vi "DFD Raised Cosine Design.vi"(4 "filtering mode":T1=2 items=["No Rate Change", "Interpolation", "Decimation"], 5 "window":u16(ring) items=["None"=0, "Hanning"=1, "Hamming"=2, "Blackman-Harris"=3, "Exact Blackman"=4, "Blackman"=5, "Flat Top"=6, "4 Term B-Harris"=7, "7 Term B-Harris"=8, "Low Sidelobe"=9, "Triangular"=30], 6 "fs in [Hz]":dbl=1.0 format="%.2f", 7 "factor":i32=2, 8 "error in (no error)":errorcluster, 9 "type":enum16{"Raised Cosine", "Root Raised Cosine"}(ring), 10 "roll off":dbl=0.2, 11 "order":i32=10) -> (0 "error out":errorcluster, 2 "order out":i32, 3 "multirate filter out":T2={"mMRate_Structure"=enum."IIR", "mMRate_Mode"=0, "mMRate_Factor"=-1, "mMRate_FIRParams"={"mMRate_FIR_H"=[], "mMRate_FIR_IsNyquist?"=FALSE, "mMRate_FIR_IsSymmetric?"=FALSE}, "mMRate_CICParams"={"mMRate_CIC_#Stage"=0, "mMRate_CIC_Lag"=0, "mMRate_CIC_Type"=enum."Lowpass"}, "mMRate_Order"=0, "mMRate_Version"="2.0", "mMRate_Comments"="", "mMRate_RationalFactor"={"mMRate_L"=-1, "mMRate_M"=-1}, "mMRate_Fs"=1.0, "mMRate_Quantized?"=FALSE, "mMRate_QFilterGain"=1.0, "mMRate_CoefWl"=16, "mMRate_Scaling"={"mMRate_ScaleByPowerOf2?"=FALSE, "mMRate_ScaleType"=enum."No Norm"}, "mMRate_InputWl"=16, "mMRate_OutputWl"=16, "mMRate_OutputMode"=enum."Truncation", "mMRate_MultMode"=enum."Truncated", "mMRate_BitPruning"=FALSE, "mMRate_GainWl"=16, "mMRate_OutputFwl"=0, "mMRate_SumIwl"=0, "mMRate_InputIwl "=16, "mMRate_SumWl"=32, "mMRate_CoefIwl"=0} {"mMRate_SumWl" min=1 max=32 step=1; "mMRate_InputIwl" min=1 max=32 step=1; "mMRate_GainWl" min=1 max=32 step=1; "mMRate_OutputWl" min=1 max=32 step=1; "mMRate_InputWl" min=1 max=32 step=1; "mMRate_CoefWl" min=1 max=32 step=1; "mMRate_Mode" items=["Default"=-1, "No Rate Change"=0, "Interpolation"=1, "Decimation"=2, "Interpolated"=3, "Rational"=4]})   [LabVIEW 2017, in "NI_DigFilterLicensed.lvlib"]
doc: "Creates a raised cosine or a root-raised cosine finite impulse response (FIR) filter."
uses:
  <vilib>/addons/Digital Filter Design/NI_DigFilterLicensed.lvlib
  <vilib>/addons/Digital Filter Design/_Objects.llb/DFD Multirate Filter Obj.ctl
  <vilib>/addons/Digital Filter Design/_Objects.llb/DFD Multirate Mode.ctl
  <vilib>/addons/Digital Filter Design/_Objects.llb/DFD Coef Norm Type.ctl
  <vilib>/addons/Digital Filter Design/_Objects.llb/DFD Round-off Mode.ctl
  <vilib>/addons/Digital Filter Design/_Objects.llb/DFD FXP MRate Multiply Mode.ctl
  <vilib>/addons/Digital Filter Design/_Objects.llb/DFD Multirate Filtering Mode.ctl
  <vilib>/addons/Digital Filter Design/FilterLib.llb/DFD Build MRate Filter from TF.vi
  <vilib>/addons/Digital Filter Design/NI_DigFilter_Process.lvlib
  <vilib>/addons/Digital Filter Design/NI_DigFilter_Design.lvlib
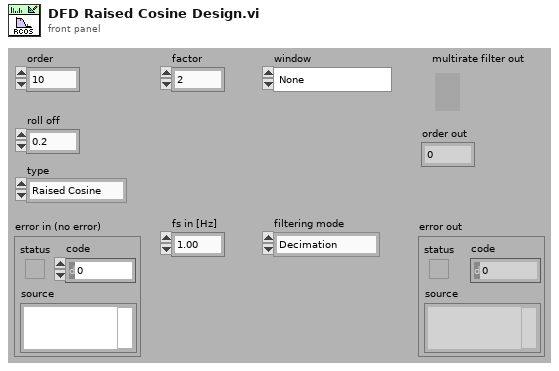
[diagram p1: front panel]
types:
  T1 = typedef "NI_DigFilterLicensed.lvlib/DFD Multirate Filtering Mode.ctl" = u16
  T2 = typedef "NI_DigFilterLicensed.lvlib/DFD Multirate Filter Obj.ctl" = cluster{"mMRate_Structure":enum16{"CIC", "FIR", "IIR", "Lattice"}, "mMRate_Mode":T3, "mMRate_Factor":i32, "mMRate_FIRParams":cluster{"mMRate_FIR_H":dbl[], "mMRate_FIR_IsNyquist?":bool, "mMRate_FIR_IsSymmetric?":bool}, "mMRate_CICParams":cluster{"mMRate_CIC_#Stage":i32, "mMRate_CIC_Lag":i32, "mMRate_CIC_Type":enum16{"Lowpass", "Highpass"}}, "mMRate_Order":i32, "mMRate_Version":string, "mMRate_Comments":string, "mMRate_RationalFactor":cluster{"mMRate_L":i32, "mMRate_M":i32}, "mMRate_Fs":dbl, "mMRate_Quantized?":bool, "mMRate_QFilterGain":dbl, "mMRate_CoefWl":i16, "mMRate_Scaling":cluster{"mMRate_ScaleByPowerOf2?":bool, "mMRate_ScaleType":T4}, "mMRate_InputWl":i16, "mMRate_OutputWl":i16, "mMRate_OutputMode":T5, "mMRate_MultMode":T6, "mMRate_BitPruning":bool, "mMRate_GainWl":i16, "mMRate_OutputFwl":i16, "mMRate_SumIwl":i16, "mMRate_InputIwl ":i16, "mMRate_SumWl":i16, "mMRate_CoefIwl":i16}
  T3 = typedef "NI_DigFilterLicensed.lvlib/DFD Multirate Mode.ctl" = i16
  T4 = typedef "NI_DigFilterLicensed.lvlib/DFD Coef Norm Type.ctl" = enum16{"No Norm", "Time Domain 1-Norm", "Time Domain 2-Norm", "Time Domain Inf-Norm"}
  T5 = typedef "NI_DigFilterLicensed.lvlib/DFD Round-off Mode.ctl" = enum16{"Nearest", "Truncation"}
  T6 = typedef "NI_DigFilterLicensed.lvlib/DFD FXP MRate Multiply Mode.ctl" = enum16{"Truncated", "Full"}
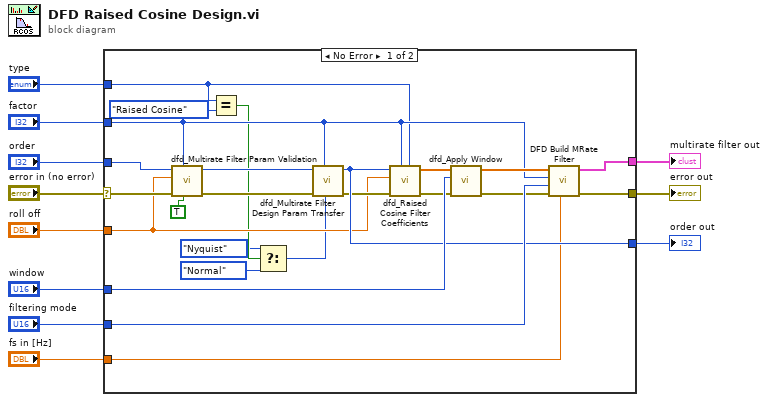
[diagram p0: block diagram]
diagram:
  n1 = case shown="No Error" "error in (no error)" {
    selector: "error in (no error)" -> [w32 w36]
    tunnel: [w33 w36] -> w11
    tunnel: [w34 _] -> w10
    tunnel: "type" -> [w14 _]
    tunnel: "order" -> [w31 _]
    tunnel: "factor" -> [w21 _]
    tunnel: "roll off" -> [w20 _]
    tunnel: "window" -> [w27 _]
    tunnel: "filtering mode" -> [w30 _]
    tunnel: [w23 _] -> w4
    tunnel: "fs in [Hz]" -> [w12 _]
    frame No Error {
      n2 = call <vilib>:"dfd_Multirate Filter Param Validation.vi"("raised cos?"=TRUE, "multirate factor"=w21, "error in (no error)"=w32, "roll off"=w20, "order"=w31) -> ("error out"=w24:errorcluster, "dup order"=w25:i32)  [unwired: 3 in, 2 out]
      n3 = Equal?(x=w14, y=enum16{"Raised Cosine", "Root Raised Cosine"}."Raised Cosine") -> (x = y?=w18:bool)
      n4 = Select(t=enum16{"Normal", "Nyquist", "Alias free"}."Nyquist" ("option"), s=w18, f=enum16{"Normal", "Nyquist", "Alias free"}."Normal" ("option")) -> (s? t:f=w15:enum16{"Normal", "Nyquist", "Alias free"})
      n5 = call <vilib>:"dfd_Multirate Filter Design Param Transfer.vi"("option"=w15, "multirate factor"=w21, "error in (no error)"=w24, "order"=w25) -> ("error out"=w22:errorcluster, "new order"=w23:i32)  [unwired: 1 in, 5 out]
      n6 = call <vilib>:"dfd_Raised Cosine Filter Coefficients.vi"("type"=w14, "#band"=w21, "error in (no error)"=w22, "roll off"=w20, "order"=w23) -> ("error out"=w26:errorcluster, "coefficients b"=w35:dbl[])  [unwired: 2 in, 3 out]
      n7 = call <vilib>:"dfd_Apply Window.vi"("error in (no error)"=w26, "window"=w27, "x"=w35) -> ("error out"=w29:errorcluster, "windowed x"=w28:dbl[])  [unwired: 1 in, 6 out]
      n8 = call-poly <vilib>:"DFD Build MRate Filter.vi"("fs in [Hz]"=w12, "error in (no error)"=w29, "filtering mode"=w30, "factor"=w21, "h(n)"=w28) -> ("error out"=w33:errorcluster, "multirate filter out"=w34:T2)  [unwired: 5 out]
    }
    frame Error {
    }
  }
  "error out" <- w11
  "multirate filter out" <- w10
  "order out" <- w4
